vi "Delete Class Genealogy.vi"   [LabVIEW 2013]
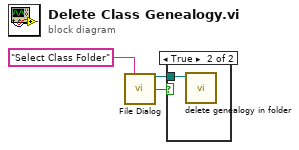
[diagram p0: block diagram]
diagram:
  n1 = call "File Dialog"("prompt"="Select Class Folder") -> ("selected path"=w3:path, "exists"=w2:bool)  [unwired: 11 in, 2 out]
  n2 = case shown="True" w2 {
    tunnel: w3 -> [_ w4]
    frame False {
    }
    frame True {
      n3 = call "delete genealogy in folder.vi"("Folder Path"=w4) -> ()  [unwired: 10 in, 1 out]
    }
  }
